vi "ModstandOgStrømUd.vi"(9 "V_out in":dbl) -> (2 "V_out out":dbl, 3 "Thermistor Modstand":dbl)   [LabVIEW 2022 SP3]
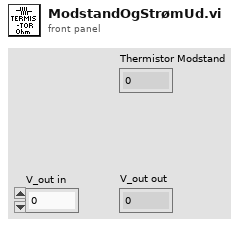
[diagram p1: front panel]
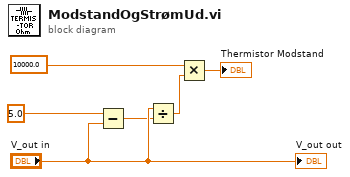
[diagram p0: block diagram]
diagram:
  n1 = Subtract(x=5.0, y="V_out in") -> (x-y=w5:dbl)
  n2 = Divide(x="V_out in", y=w5) -> (x/y=w4:dbl)
  n3 = Multiply(x=10000.0, y=w4) -> (x*y=→"Thermistor Modstand":dbl)
  "V_out out" <- "V_out in"
